vi "Build Control Setting Owner.vi"(8 "error in (no error)":errorcluster, 10 "Owner":refnum<vi>, 11 "Control Builder in":refnum<class "GUI Control Builder.lvclass">) -> (0 "error out":errorcluster, 3 "Control Builder out":refnum<class "GUI Control Builder.lvclass">)   [LabVIEW 2015, in "GUI Control Builder.lvclass"]
uses:
  GUI Control Builder.lvclass
  GUI Control Builder.lvclass/GUI Control Builder.ctl
  GUI Controls/GUI Control/GUI Control.lvclass/GUI Control.ctl
  GUI Controls/GUI Control/GUI Control.lvclass
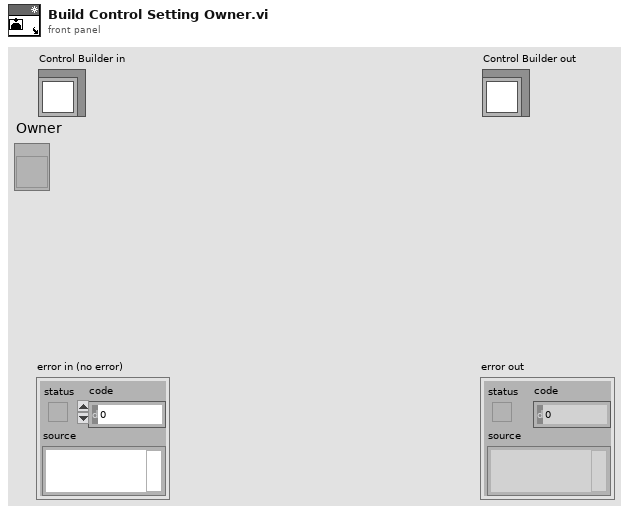
[diagram p1: front panel]
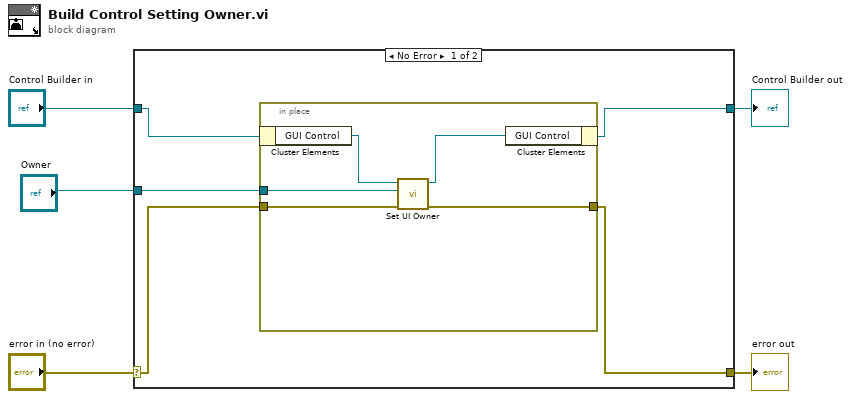
[diagram p0: block diagram]
diagram:
  n1 = case shown="No Error" "error in (no error)" {
    selector: "error in (no error)" -> [w9 w17]
    tunnel: [w7 w17] -> w4
    tunnel: [w8 w16] -> w2
    tunnel: "Control Builder in" -> [w6 w16]
    tunnel: "Owner" -> [w10 _]
    frame No Error {
      n2 = in-place {
        in-place-border: w10 -> [w15]
        in-place-border: w9 -> [w14]
        in-place-border: [w12] -> w7
        n3 = in-place-cluster #1(w6) -> ("GUI Control"=w11:refnum<class "GUI Control.lvclass">)
        n4 = call "Set UI Owner.vi"("error in (no error)"=w14, "Owner"=w15, "GUI Control"=w11) -> ("error out"=w12:errorcluster, "GUI Control out"=w13:refnum<class "GUI Control.lvclass">)  [unwired: 7 in]
        n5 = in-place-cluster #1("GUI Control"=w13) -> (w8:refnum<class "GUI Control Builder.lvclass">)
      }
    }
    frame Error {
    }
  }
  "error out" <- w4
  "Control Builder out" <- w2
